vi "DAC Configure.vi"(8 "error in":errorcluster, 11 "DAC Vacum Valve in":refnum<class "DAC Vacum Valve.lvclass">) -> (0 "error out":errorcluster, 3 "DAC Vacum Valve out":refnum<class "DAC Vacum Valve.lvclass">)   [LabVIEW 2019, in "DAC.lvlib" / "DAC Vacum Valve.lvclass"]
uses:
  DAC Vacum Valve.lvclass
  DAC.lvclass
  <vilib>/Instr/_visa.llb/VISA Configure Serial Port (Instr).vi
  C:/Users/wg/Documents/LV_Projects/test-stand/App/DAC/DAC.lvclass
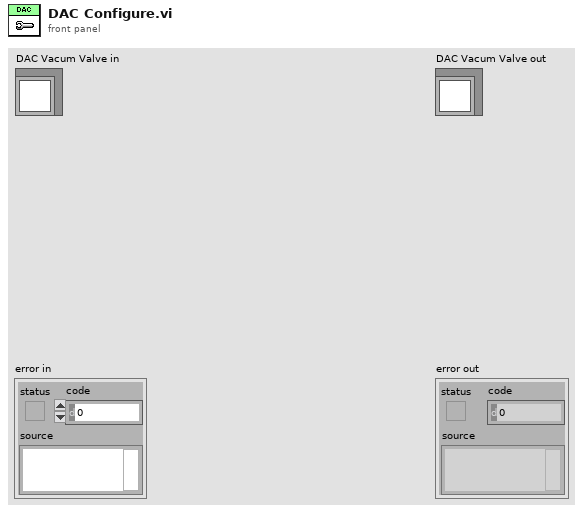
[diagram p1: front panel]
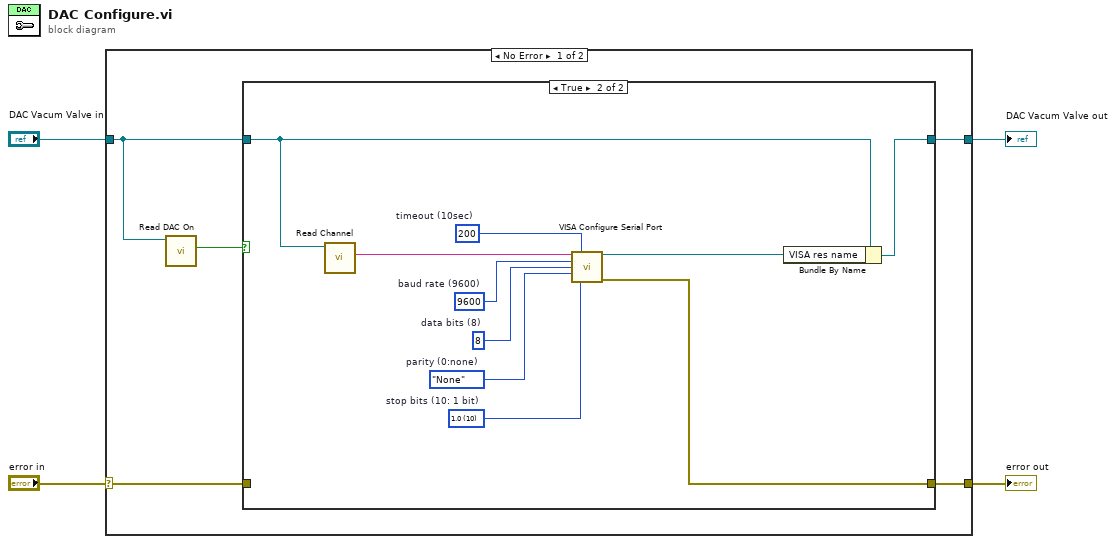
[diagram p0: block diagram]
diagram:
  n1 = case shown="No Error" "error in" {
    selector: "error in" -> [w6 w23]
    tunnel: [w5 w23] -> w4
    tunnel: [w7 w22] -> w3
    tunnel: "DAC Vacum Valve in" -> [w9 w22]
    frame No Error {
      n2 = call "Read DAC On.vi"("DAC in"=w9) -> ("DAC On"=w8:bool)  [unwired: 8 in, 2 out]
      n3 = case shown="True" w8 {
        tunnel: w9 -> [w11 w13]
        tunnel: [w11 w21] -> w7
        tunnel: w6 -> [w10 _]
        tunnel: [w10 w15] -> w5
        frame False {
          # "Temperature measurement is off."
        }
        frame True {
          w14 = u32 200  # timeout (10sec)
          w17 = u16 10 items=["1.0"=10, "1.5"=15, "2.0"=20]  # stop bits (10: 1 bit)
          w18 = enum16{"None", "Odd", "Even", "Mark", "Space"}."None"  # parity (0:none)
          w19 = u16 8  # data bits (8)
          w20 = u32 9600  # baud rate (9600)
          # "Temperature measurement is on."
          n4 = call "Read Channel.vi"("DAC in"=w13) -> ("Channel"=w12:string)  [unwired: 8 in, 2 out]
          n5 = call-poly "VISA Configure Serial Port"("VISA resource name"=w12, "timeout (10sec)"=w14, "baud rate (9600)"=w20, "data bits (8)"=w19, "parity (0:none)"=w18, "stop bits (10: 1 bit)"=w17) -> ("VISA resource name out"=w16:refnum<visa-resource-name>, "error out"=w15:errorcluster)  [unwired: 8 in]
          n6 = Bundle By Name(cluster=w13, "VISA res name"=w16) -> (w21:refnum<class "DAC Vacum Valve.lvclass">)
        }
      }
    }
    frame Error {
    }
  }
  "error out" <- w4
  "DAC Vacum Valve out" <- w3
